vi "ADAM_scan_table.vi"() -> ()   [LabVIEW 2016]
uses:
  Anemometry/Anemometry Sub Vis/Controls/Serveds.ctl
  ADAM Client/Sub VIs/ADAM Controls/Module_type_ADAM.ctl
  ADAM Client/Sub VIs/ADAM Controls/Traverse_Level_State.ctl
  Anemometry/Anemometry Sub Vis/Controls/Post_Process.ctl
  ADAM Client/Sub VIs/ADAM Controls/Channel_State.ctl
  ADAM Client/Sub VIs/ADAM Controls/Ch_description_ADAM.ctl
  ADAM Client/Sub VIs/ADAM Controls/Function_ADAM.ctl
  ADAM Client/Sub VIs/ADAM Controls/Calib_type_ADAM.ctl
  ADAM Client/Sub VIs/ADAM Controls/Address.ctl
  ADAM_Global.vi
  Sub VI's/Channel_Description_Global.vi
  Anemometry/Anemometry Sub Vis/Globals/Meas_global.vi
  Sub VI's/Logged_Data_real_Global.vi
  Anemometry/Anemometry Sub Vis/Globals/Preference_global.vi
  Anemometry/Anemometry Sub Vis/Globals/Gas_management_global.vi
  Anemometry/Anemometry Sub Vis/Globals/Constants_global.vi
panel:
  in  "Reconfigure Gills":bool
  in  "Log full Res Data":bool
  out "Duty No":u16 format="%016b"
  in  "Save Current setup":bool=TRUE
  in  "Load setup from file":bool
  out "ADAM scan comments":string
  out "History length":i32=250
  in  "stop":bool
  out "Results":dbl[](array[numeric]) format="%.3f"
  out "Titles":string[](array[string])
  # "The default value for this\nis saved in Scan_mode.txt"
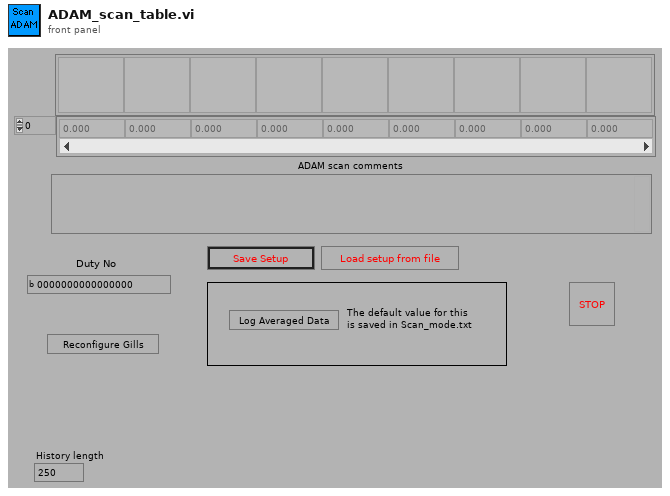
[diagram p1: front panel]
types:
  T1 = enum16{"Load ADAM setup from excel file", "Save ADAM setup to excel file"}
  T2 = typedef "Serveds.ctl" = enum16{"Read Global", "Load Global From File"}
  T3 = typedef "Module_type_ADAM.ctl" = string
  T4 = typedef "Traverse_Level_State.ctl" = enum16{"Running", "Complete"}
  T5 = typedef "Post_Process.ctl" = enum16{"Take New Data", "Post Process Raw Data File"}
  T6 = typedef "Channel_State.ctl" = enum16{"On", "Off", "Always On", "Always Off"}
  T7 = enum16{"Append to Global", "Read Global then Clear"}
  T8 = typedef "Ch_description_ADAM.ctl" = cluster{"Ch Name":string, "Type":T3, "Function":T9, "Ch State":T6, "Calibration type":T10, "A":dbl, "B":dbl, "C":dbl, "D":dbl, "Comments":string, "Address":T11, "String":string, "Duty":u16}
  T9 = typedef "Function_ADAM.ctl" = enum16{"Analogue Input", "Digital Input", "Event counter", "Event rate", "Analogue Output", "Digital Output", "Relay Output"}
  T10 = typedef "Calib_type_ADAM.ctl" = string
  T11 = typedef "Address.ctl" = cluster{"Main":i32, "Ch.":i32, "Sub":i32, "Port Name":string}
  T12 = typedef "Client_State_Cluster.ctl" = cluster{"Client Name":string, "Traverse level State":T4, "People to Email":string[], "Next Contact Time":dbl}
  T13 = typedef "LVDateTimeRec.ctl" = cluster{"fractional second":dbl, "second":i32, "minute":i32, "hour":i32, "day of month":i32, "month":i32, "year":i32, "day of week":i32, "day of year":i32, "DST":i32}
  T14 = typedef "ADAM_Comparitor.ctl" = cluster{"Ch to Monitor":string, "Channels to Kill":string, "Warn if Above":dbl, "Warn if Below":dbl, "Kill if Above":dbl, "Kill if Below":dbl, "Hysteresis Margin":dbl, "Averaging TIme (s)":dbl, "Warn Status":bool, "Kill Status":bool, "Extra Email addresses":string}
  T15 = typedef "Update_scan_value.ctl" = cluster{"Channel Name":string, "New Value":dbl}
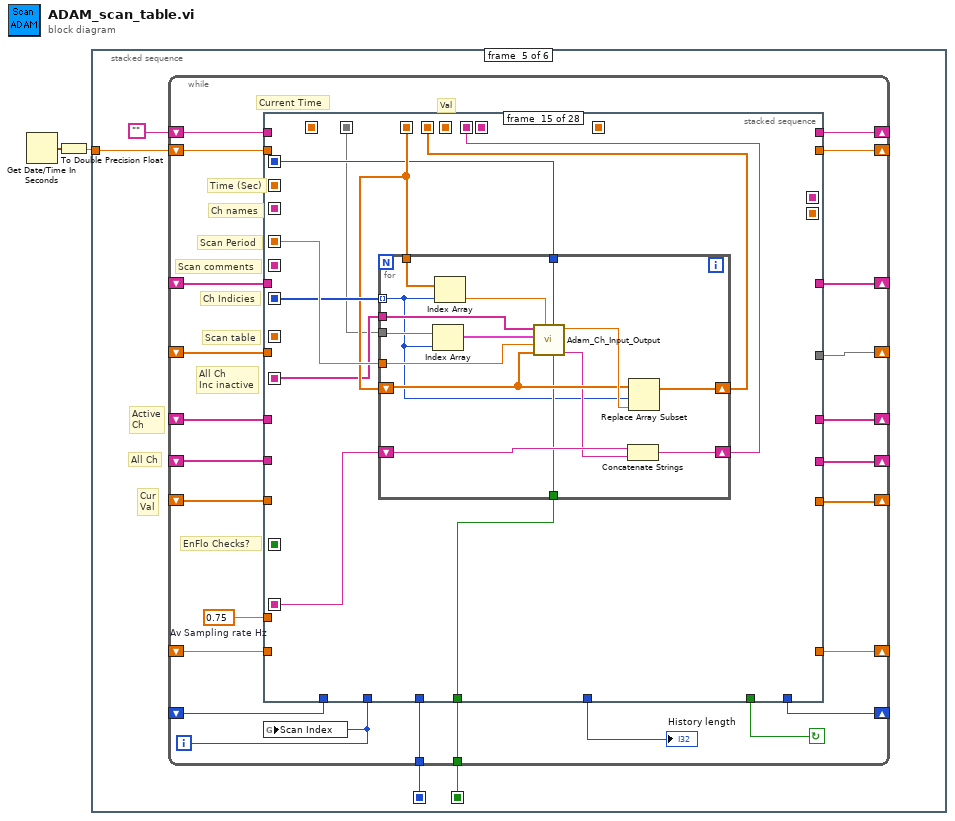
[diagram p0: block diagram]
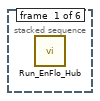
[diagram p2: hidden frame]
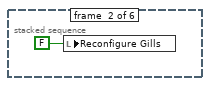
[diagram p3: hidden frame]
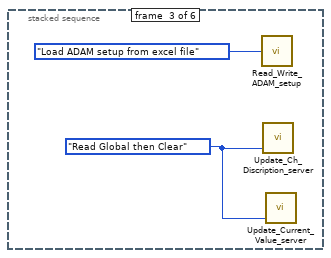
[diagram p4: hidden frame]
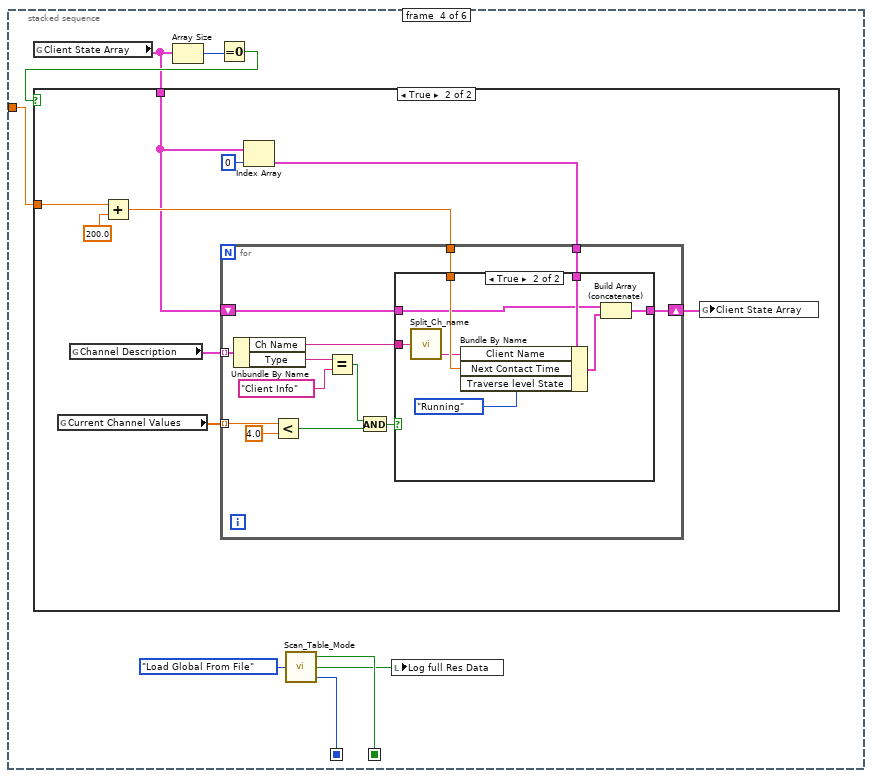
[diagram p5: hidden frame]
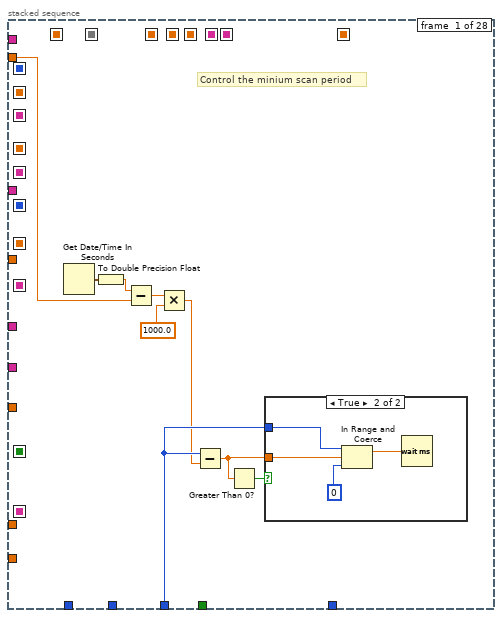
[diagram p8: hidden frame]
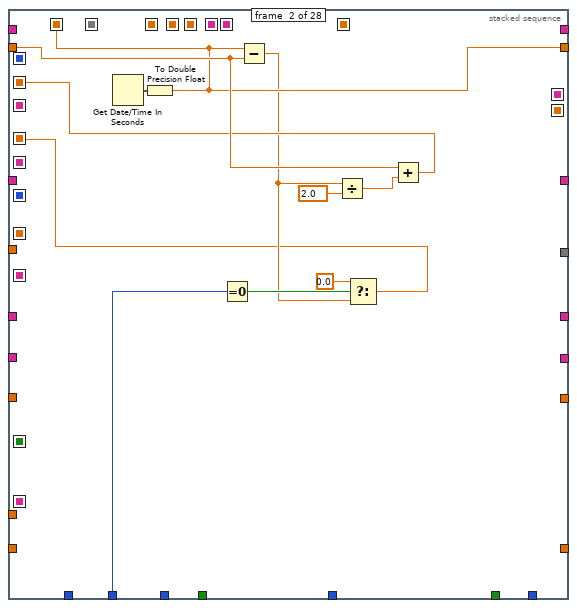
[diagram p10: hidden frame]
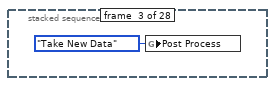
[diagram p11: hidden frame]
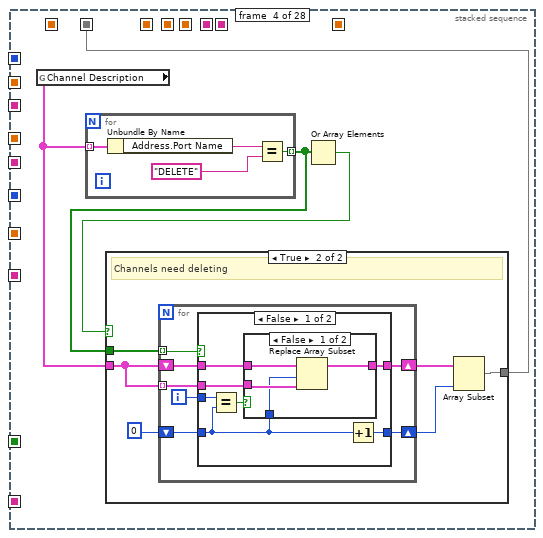
[diagram p12: hidden frame]
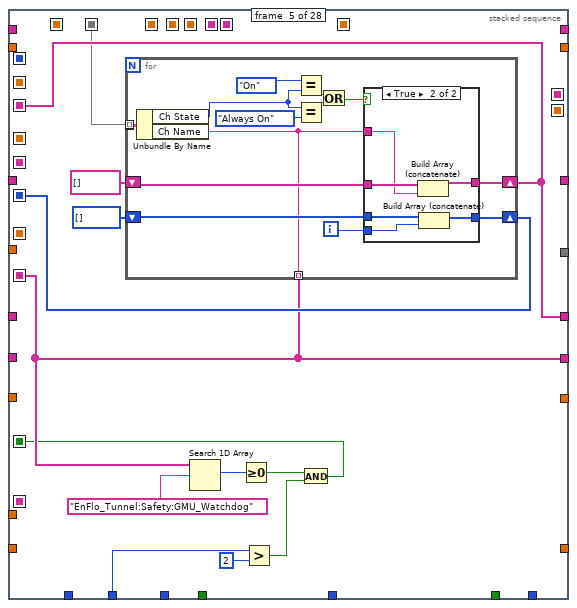
[diagram p16: hidden frame]
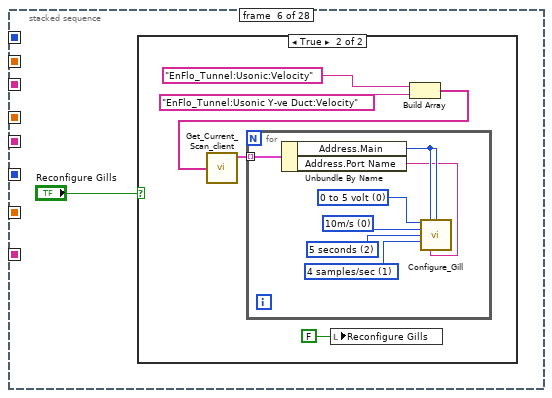
[diagram p18: hidden frame]
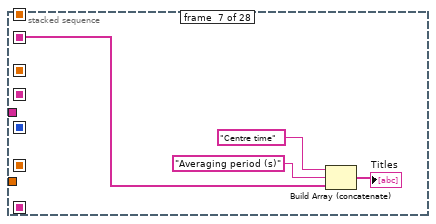
[diagram p20: hidden frame]
diagram:
  n1 = Get Date/Time In Seconds() -> (seconds since 1Jan1904=w2:timestamp)
  n2 = To Double Precision Float(number=w2) -> (double precision float=w1:dbl)
  n3 = stacked-sequence {
    seq-local: [_ _ _ w13 _ _] -> [_ _ _ _ w48 _]
    seq-local: [_ _ _ w6 _ _] -> [_ _ _ _ w45 _]
    tunnel: w1 -> [_ _ _ w8 w47 _]
    frame #0 {
      n4 = call "Run_EnFlo_Hub.vi"() -> ()  [unwired: 1 in, 7 out]
    }
    frame #1 {
      n5 = local write "Reconfigure Gills"(FALSE ("Reconfigure Gills")) -> ()
    }
    frame #2 {
      w4 = T7."Read Global then Clear" ("Mode")
      n6 = call "Read_Write_ADAM_setup.vi"("Mode"=T1."Load ADAM setup from excel file") -> ()  [unwired: 4 out]
      n7 = call "Update_Ch_Discription_server.vi"("Mode"=w4) -> ()  [unwired: 2 in, 1 out]
      n8 = call "Update_Current_Value_server.vi"("Mode"=w4) -> ()  [unwired: 2 in, 1 out]
    }
    frame #3 {
      n9 = global read "ADAM_Global.vi" "Client State Array"() -> (w9:T12[])
      n10 = Array Size(array=w9) -> (size(s)=w11:i32)
      n11 = Equal To 0?(x=w11) -> (x = 0?=w10:bool)
      n12 = case shown="True" w10 {
        tunnel: w9 -> [_ w15]
        tunnel: w8 -> [_ w18]
        frame False {
          # "No clients currently using server"
        }
        frame True {
          n13 = global read "ADAM_Global.vi" "Current Channel Values"() -> (w22:dbl[])
          n14 = global read "Channel_Description_Global.vi" "Channel Description"() -> (w21:T8[])
          n15 = Add(x=w18, y=200.0) -> (x+y=w16:dbl)
          n16 = Index Array(array=w15, index=0) -> (element=w19:T12)
          n17 = for {
            tunnel: w21 -> [w35] mode=indexing
            tunnel: w22 -> [w27] mode=indexing
            tunnel: w19 -> [w28]
            tunnel: w16 -> [w26]
            shift-right: [w25] -> w14
            shift-left: w15 -> [w24]
            n18 = Unbundle By Name(w35) -> ("Ch Name"=w23:string, "Type"=w32:T3)
            n19 = Less?(x=w27, y=4.0) -> (x < y?=w30:bool)
            n20 = Equal?(x=w32, y=T3 "Client Info" ("Type")) -> (x = y?=w31:bool)
            n21 = And(x=w31, y=w30) -> (x .and. y?=w29:bool)
            n22 = case shown="True" w29 {
              tunnel: w28 -> [_ w44]
              tunnel: w26 -> [_ w43]
              tunnel: [w36 w41] -> w25
              tunnel: w24 -> [w36 w40]
              tunnel: w23 -> [_ w38]
              frame False {
              }
              frame True {
                n23 = call "Split_Ch_name.vi"("Ch name"=w38) -> ("Low level"=w37:string)  [unwired: 2 out]
                n24 = Bundle By Name(cluster=w44, "Client Name"=w37, "Next Contact Time"=w43, "Traverse level State"=Traverse_Level_State."Running") -> (w39:T12)
                n25 = Build Array (concatenate)(w40, w39) -> (w41:T12[])
              }
            }
          }
          n26 = global write "ADAM_Global.vi" "Client State Array"(w14) -> ()
        }
      }
      n27 = call "Scan_Table_Mode.vi"("Mode"=Serveds."Load Global From File") -> ("Simulate Mode ?"=w13:bool, "Log Full Res Data?"=w7:bool, "Minimum Scan Period (ms)"=w6:i32)
      n28 = local write "Log full Res Data"(w7) -> ()
    }
    frame #4 {
      # "Active\nCh"
      # "Cur\nVal"
      # "All Ch"
      n29 = while {
        shift-left: _ -> [w57]
        shift-right: [w56] -> _
        shift-left: _ -> [w58]
        shift-right: [w59] -> _
        shift-left: _ -> [w60]
        shift-right: [w61] -> _
        tunnel: w48 -> [w62]
        shift-left: _ -> [w65]
        shift-right: [w64] -> _
        shift-left: _ -> [w66]
        shift-right: [w67] -> _
        shift-left: _ -> [w68]
        shift-right: [w69] -> _
        shift-left: w47 -> [w70]
        shift-right: [w71] -> _
        shift-right: [w54] -> _
        shift-left: _ -> [w53]
        shift-right: [w51] -> _
        shift-left: "" -> [w50]
        tunnel: w45 -> [w49]
        i -> [w52]
        stop <- w72 continue-if-true
        w55 = 0.75  # Av Sampling rate Hz
        # "Current Time"
        # "EnFlo Checks?"
        # "Val"
        # "All Ch\nInc inactive"
        # "Scan comments"
        # "Scan table"
        # "Time (Sec)"
        # "Ch Indicies"
        # "Ch names"
        # "Scan Period"
        n30 = stacked-sequence {
          seq-local: [_ _ _ _ _ _ _ _ _ _ _ _ _ _ _ _ _ _ _ w376 _ _ _ _ _ _ _ _] -> [_ _ _ _ _ _ _ _ _ _ _ _ _ _ _ _ _ _ _ _ _ w427 w432 _ _ _ w486 _]
          seq-local: [_ w93 _ _ _ _ _ _ _ _ _ _ _ _ _ _ _ _ _ _ _ _ _ _ _ _ _ _] -> [_ _ _ _ _ _ _ _ _ _ _ _ _ _ _ _ _ _ _ _ _ _ w439 _ _ _ _ _]
          seq-local: [_ _ _ _ _ _ _ w191 _ _ _ _ _ _ _ _ _ _ _ _ _ _ _ _ _ _ _ _] -> [_ _ _ _ _ _ _ _ _ w229 _ _ _ _ _ _ _ _ _ _ _ _ w437 _ _ _ _ _]
          seq-local: [_ w86 _ _ _ _ _ _ _ _ _ _ _ _ _ _ _ _ _ _ _ _ _ _ _ _ _ _] -> [_ _ _ _ _ _ _ _ _ _ _ _ _ _ w296 _ _ _ _ _ _ _ w438 _ _ _ _ _]
          seq-local: [_ _ _ _ _ _ _ w194 _ _ _ _ _ _ _ _ _ _ _ _ _ _ _ _ _ _ _ _] -> [_ _ _ _ _ _ _ _ _ w231 _ _ _ _ _ _ _ _ _ _ _ _ _ w452 _ _ _ _]
          seq-local: [_ _ _ _ _ _ _ _ _ _ _ _ _ _ w294 _ _ _ _ _ _ _ _ _ _ _ _ _] -> [_ _ _ _ _ _ _ _ _ _ _ _ _ _ _ w313 _ _ _ _ _ _ _ _ _ _ _ _]
          seq-local: [_ _ _ _ w145 _ _ _ _ _ _ _ _ _ _ _ _ _ _ _ _ _ _ _ _ _ _ _] -> [_ _ _ _ _ _ w183 w193 _ w232 w234 _ _ _ _ _ _ _ _ _ _ _ w435 _ _ _ _ _]
          seq-local: [_ _ _ _ w144 _ _ _ _ _ _ _ _ _ _ _ _ _ _ _ _ _ _ _ _ _ _ _] -> [_ _ _ _ _ _ _ _ w209 w227 _ w238 _ _ w295 _ _ _ _ _ _ _ _ _ _ _ _ _]
          seq-local: [_ _ _ _ _ _ _ w187 _ _ _ _ _ _ _ _ _ _ _ _ _ _ _ _ _ _ _ _] -> [_ _ _ _ _ _ _ _ w207 w228 _ w239 w263 _ w292 _ _ _ _ _ _ _ _ _ _ _ _ _]
          seq-local: [_ _ _ _ _ _ _ _ _ _ _ _ _ _ w290 _ _ _ _ _ _ _ _ _ _ _ _ _] -> [_ _ _ _ _ _ _ _ _ _ _ _ _ _ _ w318 w347 _ _ w374 _ _ _ _ _ _ _ _]
          seq-local: [_ _ _ _ w140 _ _ _ _ _ _ _ _ _ _ _ _ _ _ _ _ _ _ _ _ _ _ _] -> [_ _ _ _ _ _ _ w189 _ w230 _ _ _ _ w291 w317 w346 _ _ w375 w400 w419 w434 _ _ w463 _ _]
          seq-local: [_ _ _ _ _ _ _ _ _ _ _ _ _ w276 _ _ _ _ _ _ _ _ _ _ _ _ _ _] -> [_ _ _ _ _ _ _ _ _ _ _ _ _ _ w289 _ _ _ _ _ _ _ _ _ _ _ _ _]
          seq-local: [_ _ _ w98 _ _ _ _ _ _ _ _ _ _ _ _ _ _ _ _ _ _ _ _ _ _ _ _] -> [_ _ _ _ w142 _ _ _ w208 w226 _ w240 w264 _ w288 _ _ _ _ _ _ _ _ _ _ _ _ _]
          seq-local: [_ w92 _ _ _ _ _ _ _ _ _ _ _ _ _ _ _ _ _ _ _ _ _ _ _ _ _ _] -> [_ _ _ _ _ _ _ _ _ _ _ w236 w262 _ _ w314 w343 _ _ _ _ _ _ _ _ _ _ _]
          seq-local: [_ _ _ _ _ _ _ _ _ _ _ _ _ _ _ _ _ _ _ _ _ _ w431 _ _ _ _ _] -> [_ _ _ _ _ _ _ _ _ _ _ _ _ _ _ _ _ _ _ _ _ _ _ _ _ _ _ _]
          seq-local: [_ _ _ _ w134 _ _ _ _ _ _ _ _ _ _ _ _ _ _ _ _ _ _ _ _ _ _ _] -> [_ _ _ _ _ _ _ _ w216 _ w233 _ _ _ _ w316 w345 w361 _ _ _ _ _ _ _ _ _ w490]
          seq-local: [_ _ _ _ _ _ _ _ _ _ _ _ _ _ _ _ _ _ _ w373 _ _ _ _ _ _ _ _] -> [_ _ _ _ _ _ _ _ _ _ _ _ _ _ _ _ _ _ _ _ w401 _ _ _ _ _ _ _]
          seq-local: [_ _ _ _ _ _ _ _ w206 _ _ _ _ _ _ _ _ _ _ _ _ _ _ _ _ _ _ _] -> [_ _ _ _ _ _ _ _ _ _ _ _ _ _ w287 _ _ _ _ _ _ _ _ _ _ _ _ _]
          seq-local: [_ _ _ _ _ _ _ _ _ _ _ _ _ _ _ _ _ _ _ w372 _ _ _ _ _ _ _ _] -> [_ _ _ _ _ _ _ _ _ _ _ _ _ _ _ _ _ _ _ _ w399 _ _ _ _ _ _ _]
          seq-local: [_ _ _ _ _ _ _ _ _ _ _ _ _ _ _ w312 _ _ _ _ _ _ _ _ _ _ _ _] -> [_ _ _ _ _ _ _ _ _ _ _ _ _ _ _ _ _ _ _ _ _ _ _ w440 w455 _ _ _]
          tunnel: [_ _ _ _ _ _ _ _ _ _ _ _ _ _ _ _ _ _ _ _ _ _ _ _ w461 _ _ _] -> w72
          tunnel: [_ w92 _ _ _ _ _ _ _ _ _ _ _ _ _ _ _ _ _ _ _ _ _ _ _ _ _ _] -> w71
          tunnel: w70 -> [w76 w94 _ _ _ _ _ _ _ _ _ _ _ _ _ _ _ _ _ _ _ _ _ _ _ _ _ _]
          tunnel: [_ _ _ _ _ _ _ _ _ _ _ _ _ _ _ _ _ _ _ _ _ _ _ w450 _ _ _ _] -> w69
          tunnel: w68 -> [_ _ _ _ _ _ _ w194 _ _ _ _ _ _ _ _ _ _ _ _ _ _ _ _ _ _ _ _]
          tunnel: [_ _ _ _ w145 _ _ _ _ _ _ _ _ _ _ _ _ _ _ _ _ _ _ _ _ _ _ _] -> w67
          tunnel: w66 -> [_ _ _ _ _ _ _ w192 _ _ _ _ _ _ _ _ _ _ _ _ w402 _ _ _ _ _ _ _]
          tunnel: w52 -> [_ w90 _ _ w138 _ _ w190 w212 _ _ _ _ _ _ w315 _ w357 w366 _ _ _ _ _ w459 _ _ w491]
          tunnel: w65 -> [_ _ _ _ _ _ _ _ _ _ _ _ _ _ _ _ _ _ _ _ _ w425 _ _ _ _ _ _]
          tunnel: [_ _ _ _ _ _ _ _ _ _ _ _ _ _ _ _ _ _ _ _ _ w421 _ _ _ _ _ _] -> w64
          tunnel: [_ _ _ _ _ _ _ _ _ _ _ _ _ _ _ _ _ _ _ _ _ _ w436 _ _ _ _ _] -> w63
          tunnel: w62 -> [_ _ _ _ _ _ _ _ _ _ _ _ _ _ w293 _ _ _ _ _ _ _ _ _ _ _ _ _]
          tunnel: [_ _ _ _ w140 _ _ _ _ _ _ _ _ _ _ _ _ _ _ _ _ _ _ _ _ _ _ _] -> w61
          tunnel: w60 -> [_ _ _ _ _ _ _ w188 _ _ _ _ _ _ _ _ _ _ _ _ _ _ _ _ _ _ _ _]
          tunnel: [_ _ _ _ _ _ _ _ _ _ _ _ _ _ _ _ _ _ _ _ _ _ _ _ _ _ w486 _] -> w59
          tunnel: w58 -> [_ _ _ _ _ _ _ w186 _ _ _ _ _ _ _ _ _ _ _ _ _ _ _ _ _ _ _ _]
          tunnel: w57 -> [_ _ _ _ _ _ _ _ _ _ _ _ _ w277 _ _ _ _ _ _ _ _ _ _ _ _ _ _]
          tunnel: [_ _ _ _ _ _ _ _ _ _ _ _ _ w278 _ _ _ _ _ _ _ _ _ _ _ _ _ _] -> w56
          tunnel: w55 -> [_ _ _ _ _ _ _ _ w215 _ _ _ _ _ _ _ _ w360 w369 _ _ _ _ _ _ _ _ _]
          tunnel: [_ _ _ _ _ _ _ _ _ _ _ _ _ _ _ _ w344 _ _ _ _ _ _ _ _ _ _ _] -> w54
          tunnel: w53 -> [_ _ _ _ _ _ _ _ _ _ _ _ _ _ _ _ w342 _ _ _ _ _ _ _ _ _ _ _]
          tunnel: [_ _ _ _ _ _ _ _ _ _ _ _ _ _ _ _ _ _ _ _ _ _ _ _ w455 _ _ _] -> w51
          tunnel: w50 -> [_ _ _ _ _ _ _ _ _ _ _ w237 _ _ _ _ _ _ _ _ _ _ _ _ _ _ _ _]
          tunnel: w49 -> [w80 _ _ _ _ _ _ _ _ _ _ _ _ _ _ _ _ _ _ _ _ _ _ _ _ _ _ _]
          frame #0 {
            # "Control the minium scan period"
            n31 = Get Date/Time In Seconds() -> (seconds since 1Jan1904=w78:timestamp)
            n32 = To Double Precision Float(number=w78) -> (double precision float=w77:dbl)
            n33 = Subtract(x=w77, y=w76) -> (x-y=w75:dbl)
            n34 = Multiply(x=w75, y=1000.0) -> (x*y=w73:dbl)
            n35 = Subtract(x=w80, y=w73) -> (x-y=w79:dbl)
            n36 = Greater Than 0?(x=w79) -> (x > 0?=w81:bool)
            n37 = case shown="True" w81 {
              tunnel: w80 -> [_ w85]
              tunnel: w79 -> [_ w83]
              frame False {
              }
              frame True {
                n38 = In Range and Coerce(upper limit=w85, x=w83, lower limit=0) -> (coerced(x)=w82:dbl)  [unwired: 1 out]
                n39 = Wait (ms)(milliseconds to wait=w82) -> ()  [unwired: 1 out]
              }
            }
          }
          frame #1 {
            n40 = Get Date/Time In Seconds() -> (seconds since 1Jan1904=w91:timestamp)
            n41 = To Double Precision Float(number=w91) -> (double precision float=w92:dbl)
            n42 = Equal To 0?(x=w90) -> (x = 0?=w89:bool)
            n43 = Subtract(x=w92, y=w94) -> (x-y=w88:dbl)
            n44 = Divide(x=w88, y=2.0) -> (x/y=w95:dbl)
            n45 = Select(t=0.0, s=w89, f=w88) -> (s? t:f=w86:dbl)
            n46 = Add(x=w94, y=w95) -> (x+y=w93:dbl)
          }
          frame #2 {
            n47 = global write "Meas_global.vi" "Post Process"(Post_Process."Take New Data" ("Post Process")) -> ()
          }
          frame #3 {
            n48 = global read "Channel_Description_Global.vi" "Channel Description"() -> (w100:T8[])
            n49 = for {
              tunnel: w100 -> [w133] mode=indexing
              tunnel: [w130] -> w99 mode=indexing
              n50 = Unbundle By Name(w133) -> ("Address.Port Name"=w132:string)
              n51 = Equal?(x=w132, y="DELETE") -> (x = y?=w130:bool)
            }
            n52 = Or Array Elements(Boolean array=w99) -> (logical OR=w101:bool)
            n53 = case shown="True" w101 {
              tunnel: w100 -> [w102 w106]
              tunnel: w99 -> [_ w108]
              tunnel: [w102 w103] -> w98
              frame False {
                # "Nothing to delete"
              }
              frame True {
                # "Channels need deleting"
                n54 = for {
                  shift-right: [w115] -> w105
                  shift-left: w106 -> [w114]
                  tunnel: w108 -> [w110] mode=indexing
                  shift-right: [w113] -> w104
                  shift-left: 0 -> [w111]
                  tunnel: w106 -> [w112] mode=indexing
                  i -> [w109]
                  n55 = case shown="False" w110 {
                    tunnel: [w121 w129] -> w115
                    tunnel: w114 -> [w122 w129]
                    tunnel: [w119 w128] -> w113
                    tunnel: w111 -> [w118 w128]
                    tunnel: w112 -> [w120 _]
                    tunnel: w109 -> [w117 _]
                    frame False {
                      n56 = Equal?(x=w117, y=w118) -> (x = y?=w116:bool)
                      n57 = case shown="False" w116 {
                        tunnel: w122 -> [w126 w127]
                        tunnel: [w125 w127] -> w121
                        tunnel: w120 -> [w124 _]
                        tunnel: w118 -> [w123 _]
                        frame False {
                          n58 = Replace Array Subset(array=w126, new element=w124, index=w123) -> (w125:T8[])
                        }
                        frame True {
                        }
                      }
                      n59 = Increment(x=w118) -> (x+1=w119:i32)
                    }
                    frame True {
                    }
                  }
                }
                n60 = Array Subset(array=w105, length=w104) -> (w103:T8[])  [unwired: 1 in]
              }
            }
          }
          frame #4 {
            n61 = for {
              tunnel: [w159] -> _ mode=indexing
              shift-right: [w158] -> w145
              shift-left: string[] [] -> [w149]
              shift-right: [w155] -> w144
              shift-left: i32[] [] -> [w157]
              tunnel: [w147] -> w140 mode=indexing
              tunnel: w142 -> [w159] mode=indexing
              i -> [w156]
              n62 = Unbundle By Name(w159) -> ("Ch State"=w150:T6, "Ch Name"=w147:string)
              n63 = Equal?(x=Channel_State."On" ("Channel State"), y=w150) -> (x = y?=w152:bool)
              n64 = Equal?(x=w150, y=Channel_State."Always On" ("Channel State")) -> (x = y?=w151:bool)
              n65 = Or(x=w152, y=w151) -> (x .or. y?=w148:bool)
              n66 = case shown="True" w148 {
                tunnel: w149 -> [w160 w167]
                tunnel: w147 -> [_ w166]
                tunnel: [w160 w165] -> w158
                tunnel: w157 -> [w161 w164]
                tunnel: w156 -> [_ w163]
                tunnel: [w161 w162] -> w155
                frame False {
                }
                frame True {
                  n67 = Build Array (concatenate)(w167, w166) -> (w165:string[])
                  n68 = Build Array (concatenate)(w164, w163) -> (w162:i32[])
                }
              }
            }
            n69 = Search 1D Array(1D array=w140, element="EnFlo_Tunnel:Safety:GMU_Watchdog") -> (index of element=w139:i32)  [unwired: 1 out]
            n70 = Greater Or Equal To 0?(x=w139) -> (x >= 0?=w135:bool)
            n71 = Greater?(x=w138, y=2) -> (0:w136:bool)
            n72 = And(x=w135, y=w136) -> (x .and. y?=w134:bool)
          }
          frame #5 {
            n73 = case shown="True" "Reconfigure Gills" {
              frame False {
              }
              frame True {
                n74 = local write "Reconfigure Gills"(FALSE ("Reconfigure Gills")) -> ()
                n75 = Build Array("EnFlo_Tunnel:Usonic:Velocity", "EnFlo_Tunnel:Usonic Y-ve Duct:Velocity") -> (w171:string[])
                n76 = call "Get_Current_Scan_client.vi"("ADAM Ch Names"=w171) -> ("Ch Description Array"=w170:T8[])  [unwired: 3 out]
                n77 = for {
                  tunnel: w170 -> [w176] mode=indexing
                  w180 = u16 1 items=["1 sample/sec", "4 samples/sec"] ("Samples/sec")
                  w179 = u16 2 items=["OFF", "3 seconds", "5 seconds", "10 seconds"] ("Averaging Time")
                  w178 = u16 0 items=["10m/s", "20m/s", "30m/s", "40m/s", "50m/s", "60m/s", "70m/s"] ("Analogue O/P Scale")
                  w177 = u16 0 items=["0 to 5 volt", "+/-2.5 Volt", "4-20mA"] ("Analogue O/P Config")
                  n78 = Unbundle By Name(w176) -> ("Address.Main"=w175:i32, "Address.Port Name"=w174:string)
                  n79 = call "Configure_Gill.vi"("Analogue O/P Config"=w177, "ORIGINAL Address"=w175, "NEW Address"=w175, "Analogue O/P Scale"=w178, "Averaging Time"=w179, "Samples/sec"=w180, "Port Name"=w174) -> ()  [unwired: 9 out]
                }
              }
            }
          }
          frame #6 {
            n80 = Build Array (concatenate)("Centre time", "Averaging period (s)", w183) -> (→"Titles":string[])
          }
          frame #7 {
            n81 = global read "Logged_Data_real_Global.vi" "Data"() -> (w185:dbl[][])
            n82 = case shown="1, Default" w190 {
              tunnel: w185 -> [w202 w204]
              tunnel: w193 -> [w199 _]
              tunnel: w192 -> [w201 _]
              tunnel: [w200 w204] -> w191
              tunnel: w189 -> [w198 _]
              tunnel: w188 -> [w197 _]
              tunnel: [w196 w203] -> w187
              tunnel: w186 -> [w195 _]
              frame 1, Default {
                n83 = call "Check_and_edit_Scan_table.vi"("2D array input"=w202, "Original Channels"=w201, "Present Channels"=w199) -> ("2D array output"=w200:dbl[][])  [unwired: 2 out]
                n84 = call "Merge_row_DBL_values.vi"("Present Row values"=w195, "Present Channels"=w197, "Desired Channels"=w198) -> ("Desired Row values"=w196:dbl[])  [unwired: 1 out]
              }
              frame 0 {
                n85 = global read "ADAM_Global.vi" "Current Channel Values"() -> (w203:dbl[])
              }
            }
          }
          frame #8 {
            n86 = Multiply(x=w215, y=130.0) -> (x*y=w213:dbl)
            n87 = To Long Integer(number=w213) -> (32bit integer=w211:i32)
            n88 = Quotient & Remainder(x=w212, y=w211) -> (x-y*floor(x/y)=w210:i32, floor(x/y)=w205:i32)
            n89 = case shown="12" w210 {
              tunnel: w216 -> [_ _]
              tunnel: w209 -> [w223 _]
              tunnel: w208 -> [w222 _]
              tunnel: w207 -> [w221 _]
              tunnel: [w220 ""] -> w206
              tunnel: w205 -> [w218 _]
              frame 12 {
                n90 = Less?(x=w218, y=2) -> (x < y?=w219:bool)
                n91 = call "Reaffirm_ADAM_Outputs.vi"("Reset Zeros as well"=w219, "Active Ch Indicies"=w223, "Channel Description"=w222, "Current Channel Values"=w221) -> ("Scan Comments"=w224:string[])  [unwired: 2 in]
                n92 = Concatenate Strings(w224) -> (w220:string)
              }
              frame 1, Default {
              }
            }
          }
          frame #9 {
            n93 = global write "ADAM_Global.vi" "Current Channel Values"(w228) -> ()
            n94 = global write "Channel_Description_Global.vi" "Channel Description"(w226) -> ()
            n95 = global write "ADAM_Global.vi" "Active Ch names"(w232) -> ()
            n96 = global write "ADAM_Global.vi" "Scan comments"(w231) -> ()
            n97 = global write "ADAM_Global.vi" "Active Ch Indicies"(w227) -> ()
            n98 = global write "Logged_Data_real_Global.vi" "Data"(w229) -> ()
            n99 = global write "ADAM_Global.vi" "All Ch names"(w230) -> ()
          }
          frame #10 {
            n100 = case shown="True" w233 {
              tunnel: w234 -> [_ w235]
              frame False {
              }
              frame True {
                n101 = call "Gas_Status_panel.vi"("Ch names"=w235) -> ()  [unwired: 15 out]
              }
            }
          }
          frame #11 {
            n102 = case shown="True" "Log full Res Data" {
              tunnel: w238 -> [_ w249]
              tunnel: w239 -> [_ w242]
              tunnel: w236 -> [_ w245]
              tunnel: w237 -> [_ w244]
              tunnel: w240 -> [_ w243]
              frame False {
              }
              frame True {
                n103 = for {
                  tunnel: w249 -> [w251] mode=indexing
                  tunnel: w243 -> [w253]
                  tunnel: [w256] -> w248 mode=indexing
                  tunnel: [w255] -> w247 mode=indexing
                  tunnel: [w254] -> w246 mode=indexing
                  tunnel: w242 -> [w252]
                  n104 = Index Array(array=w253, index=w251) -> (element=w257:T8)
                  n105 = Index Array(array=w252, index=w251) -> (element=w250:dbl)
                  n106 = Unbundle By Name(w257) -> ("Ch Name"=w254:string, "Comments"=w256:string)
                  n107 = call "Convert_No._to_String_ADAM.vi"("Input number"=w250, "Ch Description"=w257) -> ("Output sting"=w255:string)
                }
                n108 = call "Write_Current_Row_to_log_file.vi"("Current Time"=w245, "Channel Names"=w246, "Channel Values"=w247, "Comments"=w248, "User added comment"=w244) -> ()  [unwired: 2 in, 1 out]
              }
            }
          }
          frame #12 {
            n109 = Seconds To Date/Time(time stamp (now)=w262) -> (date time rec=w261:T13)  [unwired: 1 in]
            n110 = Unbundle By Name(w261) -> ("hour"=w259:i32)
            n111 = feedback-in #1(w259) -> ()
            n112 = feedback #1() -> (w260:i32)  [unwired: 1 in]
            n113 = Not Equal?(x=w260, y=w259) -> (x != y?=w258:bool)
            n114 = case shown="True" w258 {
              tunnel: w263 -> [_ w265]
              tunnel: w262 -> [_ w267]
              tunnel: w264 -> [_ w266]
              frame False {
              }
              frame True {
                n115 = for {
                  tunnel: w266 -> [w272] mode=indexing
                  tunnel: [w275] -> w270 mode=indexing
                  tunnel: [w274] -> w269 mode=indexing
                  tunnel: [w273] -> w268 mode=indexing
                  tunnel: w265 -> [w271] mode=indexing
                  n116 = Unbundle By Name(w272) -> ("Ch Name"=w273:string, "Comments"=w275:string)
                  n117 = call "Convert_No._to_String_ADAM.vi"("Input number"=w271, "Ch Description"=w272) -> ("Output sting"=w274:string)
                }
                n118 = call "Write_All_Channels_to_Month_file.vi"("Current Time"=w267, "Channel Names"=w268, "Channel Values"=w269, "Comments"=w270) -> ()  [unwired: 3 in, 1 out]
              }
            }
          }
          frame #13 {
            n119 = Equal To 0?(x=w277) -> (x = 0?=w281:bool)
            n120 = Select(t=u16 1, s=w281, f=w277) -> (s? t:f=w276:u16)
            "Duty No" <- w276
            n121 = Equal?(x=u16 32768, y=w277) -> (x = y?=w280:bool)
            n122 = case shown="True" w280 {
              tunnel: [w283 u16 0] -> w278
              tunnel: w276 -> [w285 _]
              frame False {
                n123 = Multiply(x=u16 2, y=w285) -> (x*y=w283:u16)
              }
              frame True {
              }
            }
          }
          frame #14 {
            n124 = for {
              tunnel: w288 -> [w303]
              tunnel: w296 -> [w311]
              shift-right: [w309] -> w290
              shift-left: w292 -> [w307]
              tunnel: w291 -> [w308]
              shift-right: [w304] -> w294
              shift-left: w287 -> [w306]
              tunnel: w295 -> [w298] mode=indexing
              tunnel: w292 -> [w300]
              tunnel: w293 -> [w301]
              tunnel: w289 -> [w297]
              n125 = Index Array(array=w303, index=w298) -> (element=w302:T8)
              n126 = Index Array(array=w300, index=w298) -> (element=w299:dbl)
              n127 = call "Adam_Ch_Input_Output.vi"("Simulate"=w301, "Duty No"=w297, "Previous Scan Value"=w299, "Ch values"=w307, "Scan Period"=w311, "Ch Description"=w302, "Ch names"=w308) -> ("Scan comment"=w305:string, "Calibrated units"=w310:dbl)  [unwired: 1 in, 2 out]
              n128 = Concatenate Strings(w306, w305) -> (w304:string)
              n129 = Replace Array Subset(array=w307, new element=w310, index=w298) -> (w309:dbl[])
            }
          }
          frame #15 {
            n130 = case shown="True" w316 {
              tunnel: w318 -> [_ w325]
              tunnel: w317 -> [_ w324]
              tunnel: w315 -> [_ w323]
              tunnel: w314 -> [_ w333]
              tunnel: w313 -> [w320 w322]
              tunnel: [w320 w330] -> w312
              frame False {
              }
              frame True {
                n131 = global read "ADAM_Global.vi" "Comparitor Array"() -> (w329:T14[])
                n132 = for {
                  tunnel: w329 -> [w338] mode=indexing
                  tunnel: [w337] -> w328 mode=indexing
                  tunnel: w325 -> [w336]
                  tunnel: w324 -> [w335]
                  tunnel: [w334] -> w327 mode=indexing
                  n133 = call "ADAM_Comparitor.vi"("Comparator Info"=w338, "Ch names"=w335, "Present scan array"=w336) -> ("Comparator Info Out"=w337:T14, "Scan comment"=w334:string)  [unwired: 1 in]
                }
                n134 = call "LDA1_Safety.vi"("Adam Loop Count"=w323, "Ch Names"=w324, "Values"=w325) -> ("Scan comment"=w321:string)
                n135 = call "LDA2_Safety.vi"("Adam Loop Count"=w323, "Ch Names"=w324, "Values"=w325) -> ("Scan comment"=w326:string)
                n136 = call "Safety_Check.vi"("Adam Loop Count"=w323, "Ch Names"=w324, "Values"=w325) -> ("Scan comment"=w332:string)
                n137 = call "Check_Aero_Tunnel_on_Server.vi"("Values"=w325, "Ch Names"=w324, "Current Time"=w333, "Adam Loop Count"=w323) -> ("Scan comment"=w331:string)  [unwired: 2 in]
                n138 = global write "ADAM_Global.vi" "Comparitor Array"(w328) -> ()
                n139 = Concatenate Strings(w322, w321, w326, w332, w331, w327) -> (w330:string)
              }
            }
            n140 = property on="Results" class="Arr (strict)"() -> ("Index Values"=w319:u32[])  [unwired: 2 in, 2 out]
            n141 = property on="Titles" class="Arr (strict)"("Index Values"=w319) -> ()  [unwired: 2 in, 2 out]
          }
          frame #16 {
            n142 = Subtract(x=w343, y=w342) -> (x-y=w341:dbl)
            n143 = Greater?(x=w341, y=60.0) -> (0:w339:bool)
            n144 = case shown="True" w339 {
              tunnel: w347 -> [_ w352]
              tunnel: w346 -> [_ w351]
              tunnel: w345 -> [_ w350]
              tunnel: [w348 w349] -> w344
              tunnel: w343 -> [_ w349]
              tunnel: w342 -> [w348 _]
              frame False {
              }
              frame True {
                n145 = case shown="True" w350 {
                  tunnel: w352 -> [_ w354]
                  tunnel: w351 -> [_ w353]
                  frame False {
                  }
                  frame True {
                    n146 = call "Do_Every_minute.vi"("Ch Names"=w353, "Values"=w354) -> ()  [unwired: 1 out]
                  }
                }
              }
            }
          }
          frame #17 {
            n147 = Multiply(x=w360, y=350.0) -> (x*y=w358:dbl)
            n148 = To Long Integer(number=w358) -> (32bit integer=w356:i32)
            n149 = Quotient & Remainder(x=w357, y=w356) -> (x-y*floor(x/y)=w355:i32)  [unwired: 1 out]
            n150 = case shown="0" w355 {
              tunnel: w361 -> [w362 _]
              frame 0 {
                n151 = case shown="True" w362 {
                  frame False {
                  }
                  frame True {
                    w363 = TRUE  # Set Watchdogs
                    n152 = call "Set_Adam_Watchdogs.vi"("Set Watchdogs"=w363) -> ()  [unwired: 1 out]
                  }
                }
              }
              frame 1, Default {
              }
            }
          }
          frame #18 {
            n153 = Multiply(x=w369, y=55.0) -> (x*y=w367:dbl)
            n154 = To Long Integer(number=w367) -> (32bit integer=w365:i32)
            n155 = Quotient & Remainder(x=w366, y=w365) -> (x-y*floor(x/y)=w364:i32)  [unwired: 1 out]
            n156 = case shown="0" w364 {
              frame 0 {
                n157 = case shown="True" "Save Current setup" {
                  frame False {
                  }
                  frame True {
                    n158 = call "Read_Write_ADAM_setup.vi"("Mode"=T1."Save ADAM setup to excel file") -> ()  [unwired: 4 out]
                  }
                }
              }
              frame 1, Default {
              }
            }
          }
          frame #19 {
            n159 = call "Update_Current_Value_server.vi"("Mode"=T7."Read Global then Clear") -> ("Update array out"=w378:T15[])  [unwired: 2 in]
            n160 = for {
              tunnel: w375 -> [w386]
              tunnel: w378 -> [w381] mode=indexing
              shift-right: [w384] -> w376
              shift-left: w374 -> [w385]
              tunnel: [w380] -> w373 mode=indexing
              tunnel: [w379] -> w372 mode=indexing
              n161 = Unbundle By Name(w381) -> ("Channel Name"=w380:string, "New Value"=w379:dbl)
              n162 = Search 1D Array(1D array=w386, element=w380) -> (index of element=w383:i32)  [unwired: 1 out]
              n163 = Less Than 0?(x=w383) -> (x < 0?=w382:bool)
              n164 = case shown="True" w382 {
                tunnel: w380 -> [_ w387]
                tunnel: w381 -> [_ w392]
                frame False {
                }
                frame True {
                  n165 = call "Check_Ch_Name_colons.vi"("No of Colons"=2, "Ch Name in"=w387) -> ("Ch Name out"=w388:string)
                  n166 = global read "ADAM_Global.vi" "Update Current Value"() -> (w391:T15[])
                  n167 = Bundle By Name(cluster=T8 {"Ch Name"="", "Type"="Hold Value", "Function"=enum."Analogue Input", "Ch State"=enum."On", "Calibration type"="", "A"=0.0, "B"=0.0, "C"=0.0, "D"=0.0, "Comments"="", "Address"={"Main"=0, "Ch."=0, "Sub"=0, "Port Name"=""}, "String"="", "Duty"=0} ("Ch Description"), "Ch Name"=w388, "Type"=T3 "Hold Value") -> (w396:T8)
                  n168 = Build Array (concatenate)(w391, w392) -> (w390:T15[])
                  n169 = global read "Preference_global.vi" "Rig Setup"() -> (w394:string)
                  n170 = global write "ADAM_Global.vi" "Update Current Value"(w390) -> ()
                  n171 = Build Array(w396) -> (w395:T8[])
                  n172 = call "Update_Ch_Discription_server.vi"("Mode"=T7."Append to Global", "Client HD name"=w394, "Channels to update In"=w395) -> ()  [unwired: 1 out]
                }
              }
              n173 = Replace Array Subset(array=w385, new element=w379, index=w383) -> (w384:dbl[])
            }
          }
          frame #20 {
            n174 = for {
              tunnel: w402 -> [w410]
              tunnel: w401 -> [w408] mode=indexing
              tunnel: w400 -> [w409]
              tunnel: w399 -> [w406] mode=indexing
              n175 = Search 1D Array(1D array=w410, element=w408) -> (index of element=w407:i32)  [unwired: 1 out]
              n176 = Not Equal To 0?(x=w406) -> (x != 0?=w404:bool)
              n177 = Less Than 0?(x=w407) -> (x < 0?=w405:bool)
              n178 = And(x=w404, y=w405) -> (x .and. y?=w403:bool)
              n179 = case shown="True" w403 {
                tunnel: w409 -> [_ w418]
                tunnel: w408 -> [_ w417]
                frame False {
                }
                frame True {
                  n180 = global read "Channel_Description_Global.vi" "Channel Description"() -> (w413:T8[])
                  n181 = Search 1D Array(1D array=w418, element=w417) -> (index of element=w412:i32)  [unwired: 1 out]
                  n182 = Index Array(array=w413, index=w412) -> (element=w416:T8)
                  n183 = Bundle By Name(cluster=w416, "Ch State"=Channel_State."On") -> (w414:T8)
                  n184 = Replace Array Subset(array=w413, new element=w414, index=w412) -> (w411:T8[])
                  n185 = global write "Channel_Description_Global.vi" "Channel Description"(w411) -> ()
                }
              }
            }
          }
          frame #21 {
            n186 = Search 1D Array(1D array=w419, element="GMU:Source:Release Temp") -> (index of element=w426:i32)  [unwired: 1 out]
            n187 = Index Array(array=w427, index=w426) -> (element=w424:dbl)
            n188 = Build Array (concatenate)(w424, w425) -> (w423:dbl[])
            n189 = Array Subset(array=w423, length=10 ("Array Length")) -> (w421:dbl[])  [unwired: 1 in]
            n190 = call "Mean_fr_NaN_data.vi"("Data"=w421) -> ("Mean value"=w420:dbl)  [unwired: 1 out]
            n191 = global write "Gas_management_global.vi" "Release temp (deg C)"(w420) -> ()
          }
          frame #22 {
            w429 = 500000  # Table size
            # "#HereItIs The magic number setting the ADAM table size"
            n192 = call "Merge_row_DBL_values.vi"("Present Row values"=w432, "Present Channels"=w434, "Desired Channels"=w435) -> ("Desired Row values"=w433:dbl[])  [unwired: 1 out]
            n193 = Build Array (concatenate)(w439, w438, w433) -> (w431:dbl[])
            "Results" <- w431
            n194 = call "Manipulate_Table.vi"("Table size"=w429, "Latest Row"=w431, "Table Input"=w437) -> ("History length"=w436:i32, "Table Output"=w430:dbl[][])  [unwired: 1 out]
            n195 = global write "Logged_Data_real_Global.vi" "Data"(w430) -> ()
          }
          frame #23 {
            w448 = 150 ("length")
            w449 = 50  # History length
            n196 = String Subset(string=w440, length (rest)=w448) -> (substring=w442:string)  [unwired: 1 out]
            n197 = String Length(string=w442) -> (length=w447:i32)
            n198 = Equal?(x=w448, y=w447) -> (x = y?=w446:bool)
            n199 = Select(t=" Clipped ", s=w446, f="") -> (s? t:f=w443:string)
            n200 = Concatenate Strings(w443, w442) -> (w441:string)
            n201 = Build Array (concatenate)(w452, w441) -> (w451:string[])
            n202 = Array Size(array=w451) -> (size(s)=w454:i32)
            n203 = Subtract(x=w454, y=w449) -> (x-y=w453:i32)
            n204 = Array Subset(array=w451, index=w453) -> (w450:string[])  [unwired: 1 in]
            "ADAM scan comments" <- w440
          }
          frame #24 {
            n205 = Format Into String(format string="%s %d %s" ("Format String"), "\nScan No " ("Header message"), w459, "\n") -> (resulting string=w458:string)  [unwired: 2 in, 1 out]
            n206 = call "Write_out_serial_log.vi"("Header message"=w458) -> ()
            n207 = Not(x="stop") -> (.not. x?=w461:bool)
          }
          frame #25 {
            n208 = call "Update_Ch_Discription_server.vi"("Mode"=T7."Read Global then Clear") -> ("Channels to update Out"=w464:T8[])  [unwired: 2 in]
            n209 = Array Size(array=w464) -> (size(s)=w466:i32)
            n210 = Equal To 0?(x=w466) -> (x = 0?=w465:bool)
            n211 = case shown="False" w465 {
              tunnel: w463 -> [w471 _]
              tunnel: w464 -> [w470 _]
              frame False {
                n212 = global read "Channel_Description_Global.vi" "Channel Description"() -> (w469:T8[])
                n213 = for {
                  tunnel: w471 -> [w478]
                  tunnel: w470 -> [w475] mode=indexing
                  shift-right: [w474] -> w468
                  shift-left: w469 -> [w477]
                  n214 = Unbundle By Name(w475) -> ("Ch Name"=w476:string)
                  n215 = Search 1D Array(1D array=w478, element=w476) -> (index of element=w472:i32)  [unwired: 1 out]
                  n216 = Less Than 0?(x=w472) -> (x < 0?=w473:bool)
                  n217 = case shown="False" w473 {
                    tunnel: w477 -> [w482 w485]
                    tunnel: w475 -> [w481 w483]
                    tunnel: [w480 w484] -> w474
                    tunnel: w472 -> [w479 _]
                    frame False {
                      n218 = Replace Array Subset(array=w482, new element=w481, index=w479) -> (w480:T8[])
                    }
                    frame True {
                      n219 = Build Array (concatenate)(w485, w483) -> (w484:T8[])
                    }
                  }
                }
                n220 = global write "Channel_Description_Global.vi" "Channel Description"(w468) -> ()
              }
              frame True {
              }
            }
          }
          frame #26 {
            n221 = case shown="True" "Load setup from file" {
              frame False {
              }
              frame True {
                n222 = local write "Save Current setup"(TRUE ("Save Current setup")) -> ()
                n223 = call "Read_Write_ADAM_setup.vi"("Mode"=T1."Load ADAM setup from excel file") -> ()  [unwired: 4 out]
              }
            }
          }
          frame #27 {
            n224 = case shown="0" w491 {
              tunnel: w490 -> [_ _]
              frame 0 {
                n225 = global read "Constants_global.vi" "EnFlo SW Folder"() -> (w496:path)
                n226 = Build Path(base path=w496, name or relative path=path "ADAM Client/ADAM client VIs/Plot_Server_Data.vi") -> (appended path=w493:path)
                n227 = call "Load_Comparitor_Cluster.vi"() -> ()  [unwired: 12 in]
                n228 = Build Path(base path=w496, name or relative path=path "ADAM Server/Log_ADAM_scan_table.vi") -> (appended path=w494:path)
                n229 = Build Array(w494, w493) -> (w492:path[])
                n230 = for {
                  tunnel: w492 -> [w498] mode=indexing
                  n231 = Open VI Reference(vi path=w498) -> (vi reference=w502:refnum<vi>, error out=w501:errorcluster)  [unwired: 2 in, 3 out]
                  n232 = property class="VI"(reference=w502, error in=w501, "Front Panel Window:Open"=TRUE) -> (reference out=w499:refnum<vi>, error out=w500:errorcluster)
                  n233 = invoke class="VI" method="Run VI"(reference=w499, error in=w500, "Wait until done"=FALSE) -> (reference out=w506:refnum<vi>, error out=w505:errorcluster)  [unwired: 2 in, 3 out]
                  n234 = Close Reference(reference=w506, error in (no error)=w505) -> ()  [unwired: 1 out]
                }
              }
              frame 1, Default {
              }
            }
          }
        }
        "History length" <- w63
        n235 = global write "ADAM_Global.vi" "Scan Index"(w52) -> ()
      }
    }
    frame #5 {
      w507 = FALSE  # Set Watchdogs
      n236 = call "Set_Adam_Watchdogs.vi"("Set Watchdogs"=w507) -> ()  [unwired: 1 out]
      n237 = call "Read_Write_ADAM_setup.vi"("Mode"=T1."Save ADAM setup to excel file") -> ()  [unwired: 4 out]
    }
  }
